vi "Z_Hswich_prop.vi"(8 "error in (no error)":errorcluster, 9 "source":T1, 10 "connect":bool, 11 "Control":refnum<vi>) -> (0 "error our":errorcluster)   [LabVIEW 2019]
uses:
  Z_Hswitch.xctl
  Y_source.ctl
  Trigers/D^.vi
  Timer Delay/Timer.vi
  Counter/Counter.lvlib
  Logik/Logik.lvlib
  Heating.lvlib
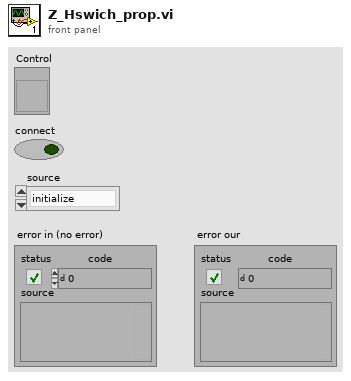
[diagram p1: front panel]
types:
  T1 = typedef "Heating.lvlib/Y_source.ctl" = enum8{"initialize", "local disabled", "local hand", "hand", "auto", "dist"}
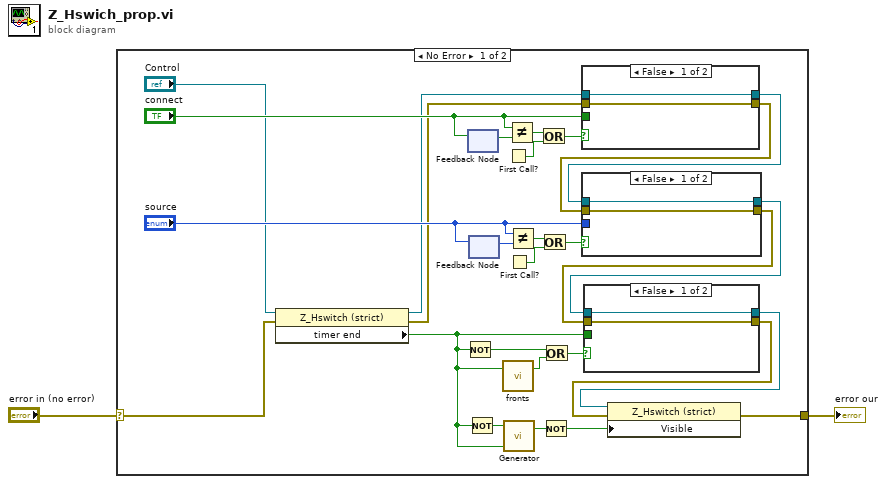
[diagram p0: block diagram]
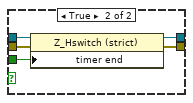
[diagram p2: hidden frame]
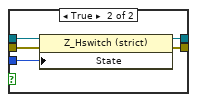
[diagram p3: hidden frame]
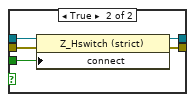
[diagram p4: hidden frame]
diagram:
  n1 = case shown="No Error" "error in (no error)" {
    selector: "error in (no error)" -> [w3 w52]
    tunnel: [w4 w52] -> w2
    frame No Error {
      n2 = property on="Property Node" class="Z_Hswitch (strict)"(reference="Control", error in=w3) -> (reference out=w12:refnum<vi>, error out=w8:errorcluster, "timer end"=w14:bool)
      n3 = Not(x=w14) -> (.not. x?=w16:bool)
      n4 = Not(x=w14) -> (.not. x?=w15:bool)
      n5 = feedback #1() -> (w27:bool)  [unwired: 1 in]
      n6 = feedback-in #1("connect") -> ()
      n7 = feedback #2() -> (w23:T1)  [unwired: 1 in]
      n8 = feedback-in #2("source") -> ()
      n9 = call "fronts.vi"("in"=w14) -> ("raise"=w17:bool)  [unwired: 1 in, 1 out]
      n10 = First Call?() -> (First Call?: T/F=w28:bool)
      n11 = call "Generator.vi"("R"=w14, "ON (F)"=w15) -> ("Q"=w19:bool)  [unwired: 2 in]
      n12 = First Call?() -> (First Call?: T/F=w25:bool)
      n13 = Not Equal?(x="connect", y=w27) -> (x != y?=w26:bool)
      n14 = Not Equal?(x="source", y=w23) -> (x != y?=w22:bool)
      n15 = Or(x=w26, y=w28) -> (x .or. y?=w29:bool)
      n16 = Or(x=w22, y=w25) -> (x .or. y?=w24:bool)
      n17 = Not(x=w19) -> (.not. x?=w20:bool)
      n18 = Or(x=w16, y=w17) -> (x .or. y?=w18:bool)
      n19 = case shown="False" w29 {
        tunnel: "connect" -> [_ w51]
        tunnel: w12 -> [w46 w50]
        tunnel: [w46 w49] -> w11
        tunnel: w8 -> [w45 w48]
        tunnel: [w45 w47] -> w7
        frame False {
        }
        frame True {
          n20 = property on="Property Node" class="Z_Hswitch (strict)"(reference=w50, error in=w48, "connect"=w51) -> (reference out=w49:refnum<vi>, error out=w47:errorcluster)
        }
      }
      n21 = case shown="False" w24 {
        tunnel: "source" -> [_ w43]
        tunnel: w11 -> [w39 w44]
        tunnel: [w39 w42] -> w10
        tunnel: w7 -> [w38 w41]
        tunnel: [w38 w40] -> w6
        frame False {
        }
        frame True {
          n22 = property on="Property Node" class="Z_Hswitch (strict)"(reference=w44, error in=w41, "State"=w43) -> (reference out=w42:refnum<vi>, error out=w40:errorcluster)
        }
      }
      n23 = case shown="False" w18 {
        tunnel: w14 -> [_ w37]
        tunnel: w10 -> [w32 w36]
        tunnel: [w32 w35] -> w9
        tunnel: w6 -> [w31 w34]
        tunnel: [w31 w33] -> w5
        frame False {
        }
        frame True {
          n24 = property on="Property Node" class="Z_Hswitch (strict)"(reference=w36, error in=w34, "timer end"=w37) -> (reference out=w35:refnum<vi>, error out=w33:errorcluster)
        }
      }
      n25 = property on="Property Node" class="Z_Hswitch (strict)"(reference=w9, error in=w5, "Visible"=w20) -> (error out=w4:errorcluster)  [unwired: 1 out]
    }
    frame Error {
    }
  }
  "error our" <- w2
